vi "loadExcelAssignData.vi"() -> ()   [LabVIEW 2012]
panel:
  out "appended path":path
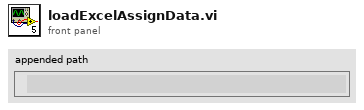
[diagram p1: front panel]
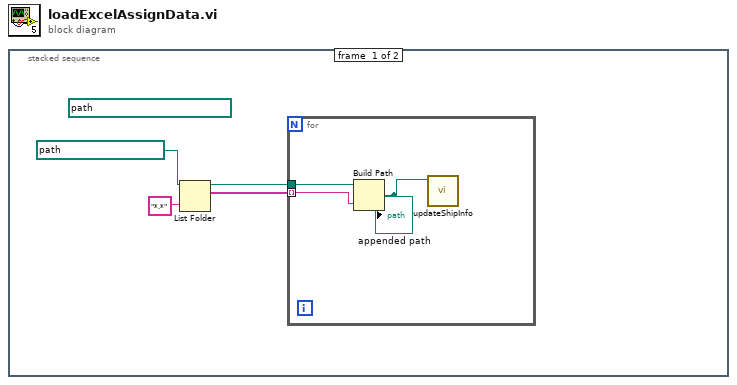
[diagram p0: block diagram]
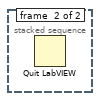
[diagram p2: hidden frame]
diagram:
  n1 = stacked-sequence {
    frame #0 {
      (unwired) path "o:/monitor/回貨明細/temp" ("path")
      n2 = List Folder(path=path "o:/monitor/回貨明細", pattern="*.*") -> (path out=w3:path, filenames=w2:string[])  [unwired: 2 in, 2 out]
      n3 = for {
        tunnel: w3 -> [w7]
        tunnel: w2 -> [w6] mode=indexing
        n4 = Build Path(base path=w7, name or relative path=w6) -> (appended path=w5:path)
        "appended path" <- w5
        n5 = call "updateShipInfo.vi"("template (empty)"=w5) -> ()  [unwired: 11 in]
      }
    }
    frame #1 {
      n6 = Quit LabVIEW() -> ()  [unwired: 1 in]
    }
  }
